vi "libera.vi"() -> ()   [LabVIEW 2014]
uses:
  chaos-common-crest/LabVIEW/LV14/chaosui-crest/VIs/ChaosDevState.ctl
  <vilib>/Utility/file.llb/Write To Spreadsheet File (I64).vi
  chaos-common-crest/LabVIEW/LV14/chaosui-crest/chaosui-crest.lvlib
panel:
  in  "DataFile":path
  out "libera_error":i32
  out "STATUS":string
  out "SA_OUT":T1(array[cluster])
  out "ADC_CW":T2(array[cluster])
  out "AVG_OUT":cluster{"AVG":i32}[](array[cluster])
  out "ADC_SP":T3(array[cluster])
  in  "AVG":bool=TRUE
  in  "STATE":bool=TRUE
  in  "stop":bool
  in  "loops":i32=10
  in  "DECIMATED":bool
  out "DD_OUT":T4(array[cluster])
  in  "refresh (ms)":u32=200
  out "samples":i32
  out "mode":i32
  out "Device State":T5
  out "nok":i32
  out "dev_error":bool
  out "acquisitions":u64
  out "timestamp":u64
  in  "Samples":u32=10
  in  "TRIGGERED":bool
  in  "ADC CW":bool
  in  "ADC SP":bool
  in  "SA":bool
  in  "DD":bool
  in  "!CHAOS URL":string="chaost-webui1.chaos.lnf.infn.it:8081"
  in  "LiberaID":string="LIBERA02/LIBERA_ACQUIRE0"
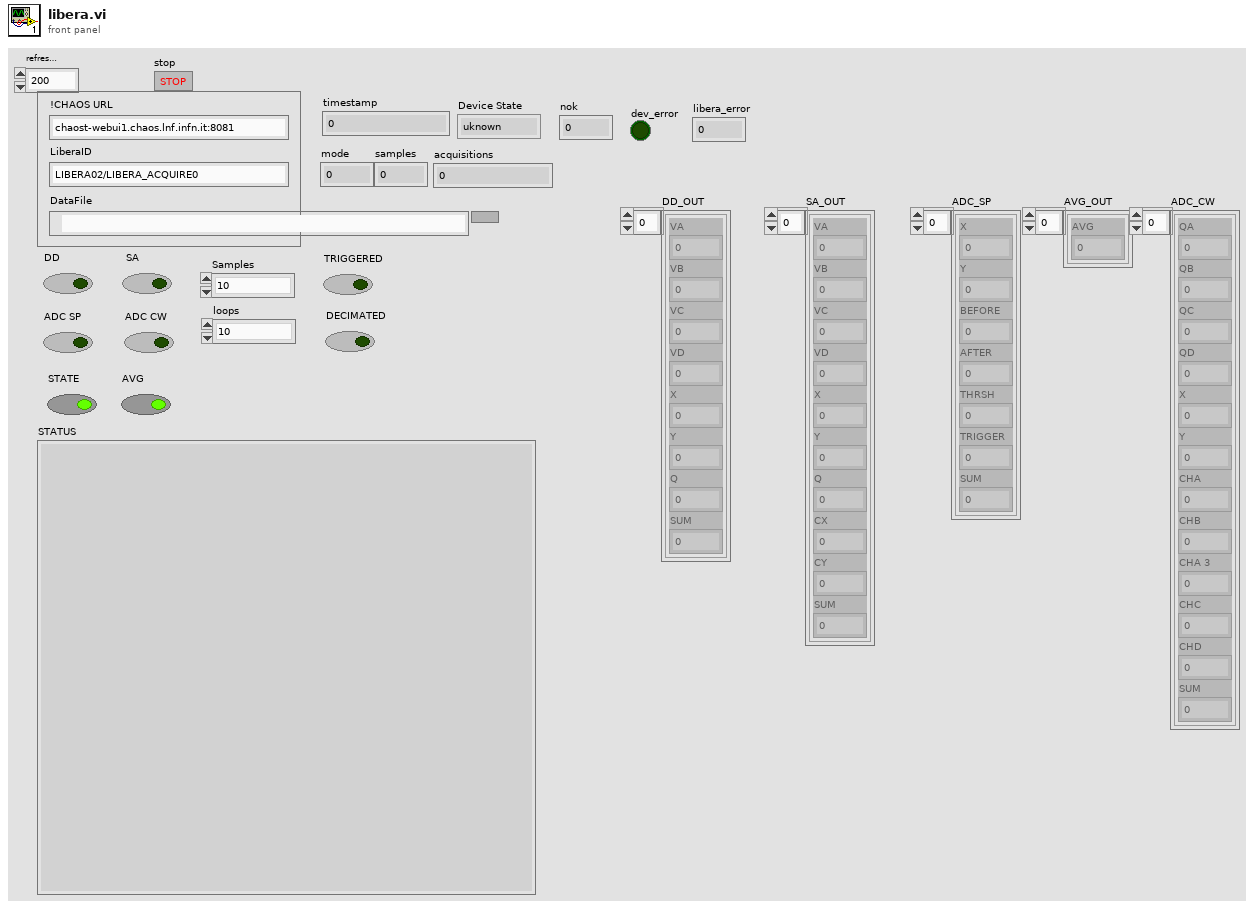
[diagram p1: front panel]
types:
  T1 = cluster{"VA":i32, "VB":i32, "VC":i32, "VD":i32, "X":i32, "Y ":i32, "Q":i32, "CX":i32, "CY":i32, "SUM":i32}[]
  T2 = cluster{"QA":i32, "QB":i32, "QC":i32, "QD":i32, "X":i32, "Y":i32, "CHA":i32, "CHB":i32, "CHA 3":i32, "CHC":i32, "CHD":i32, "SUM":i32}[]
  T3 = cluster{"X":i32, "Y":i32, "BEFORE":i32, "AFTER":i32, "THRSH":i32, "TRIGGER":i32, "SUM":i32}[]
  T4 = cluster{"VA":i32, "VB":i32, "VC":i32, "VD":i32, "X":i32, "Y ":i32, "Q":i32, "SUM":i32}[]
  T5 = typedef "ChaosDevState.ctl" = enum16{"uknown", "stop", "init", "deinit", "start"}
  T6 = typedef "LabVIEWHTTPClient.lvlib/ClientHandle.ctl" = refnum<k1>
  T7 = cluster{"client handle out":T6, "chaoswanurl":string}
  T8 = enum16{"stopAcquire", "setTime", "acquireAVG", "acquireADCSP", "acquireADCCW", "acquireStream", "acquireDD"}
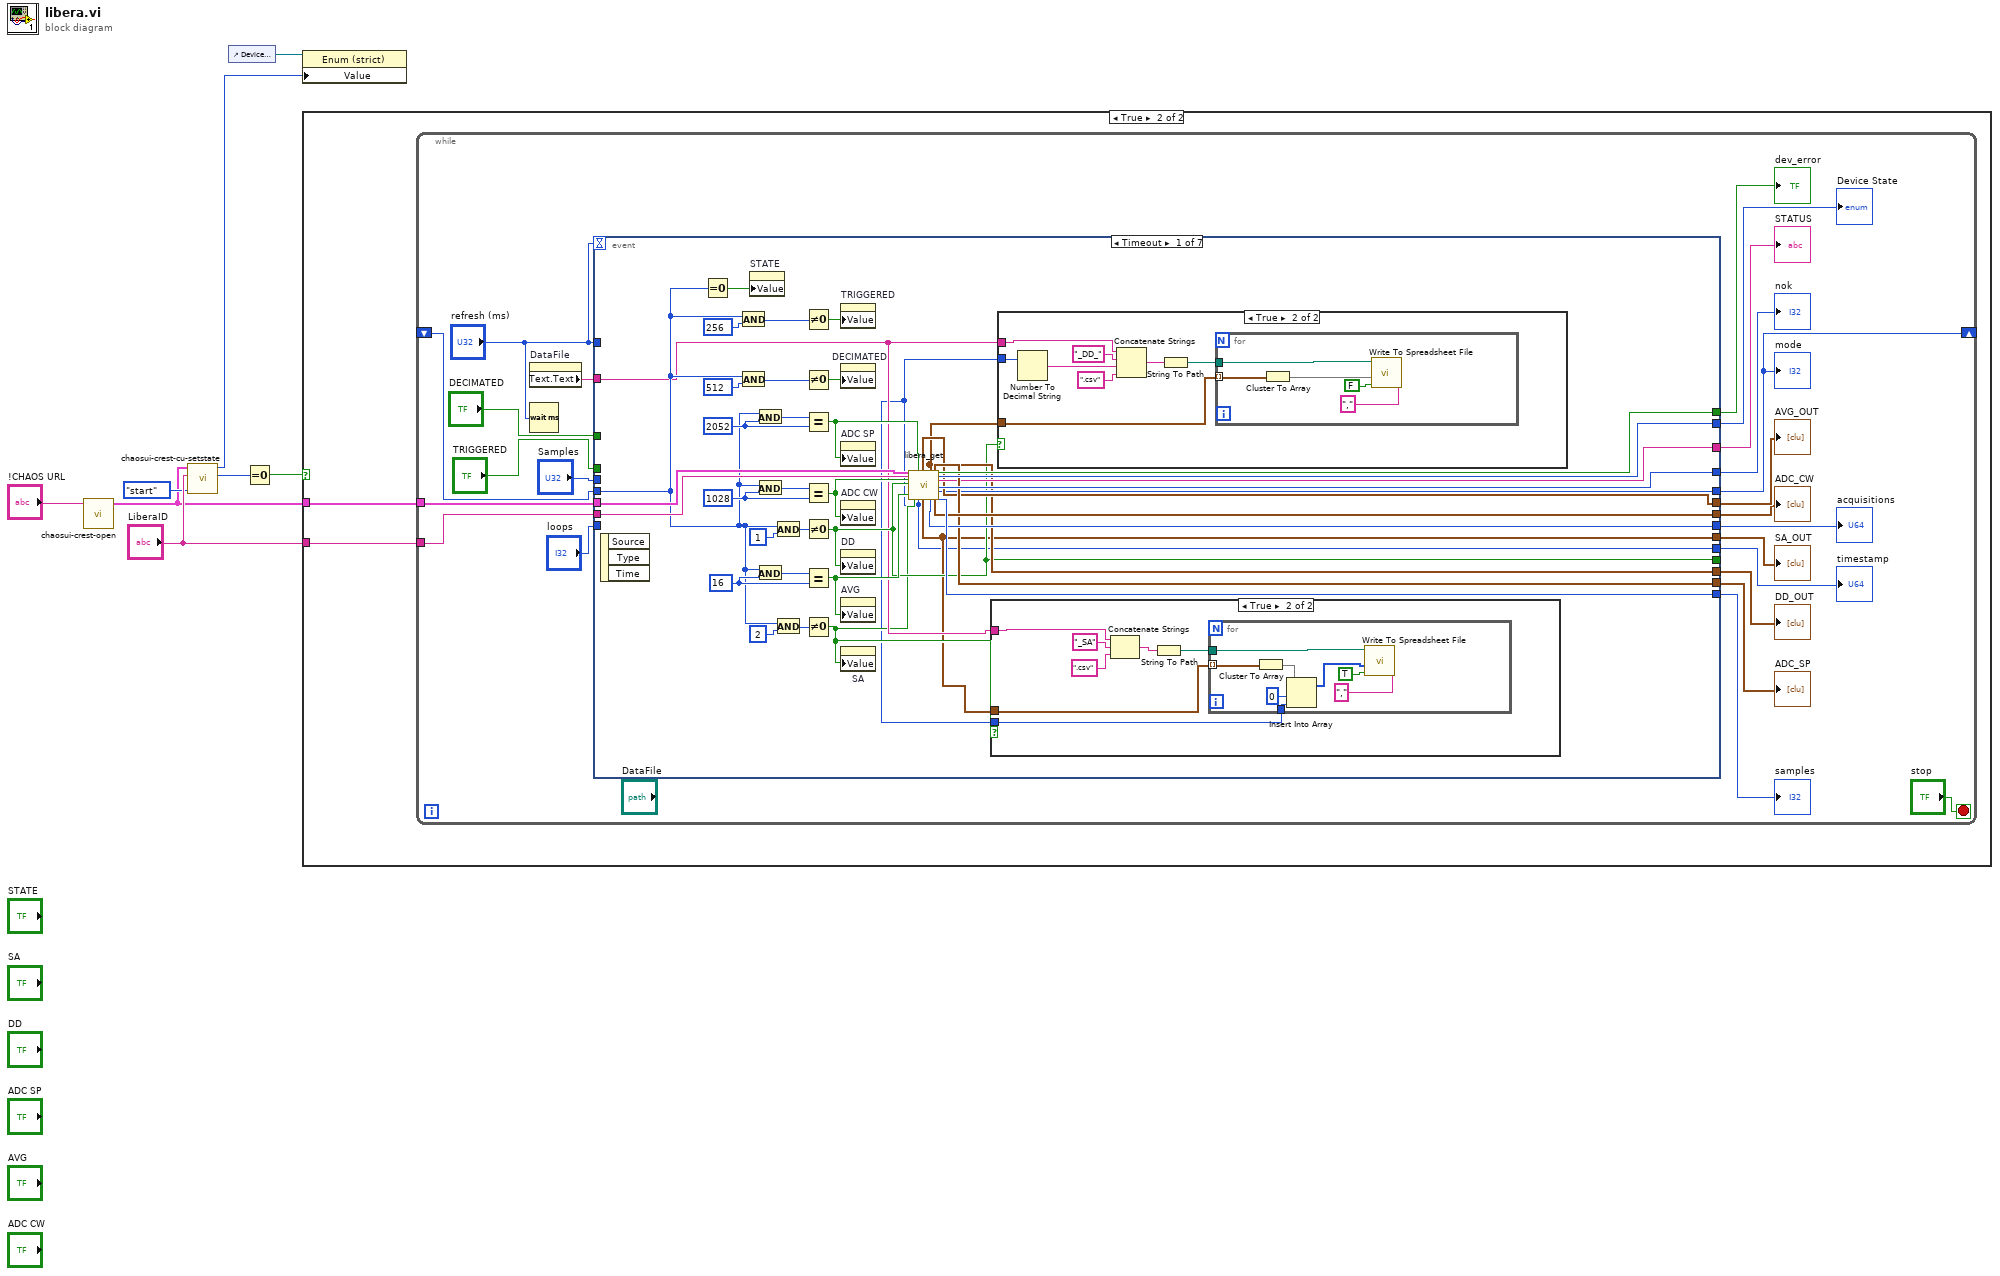
[diagram p0: block diagram]
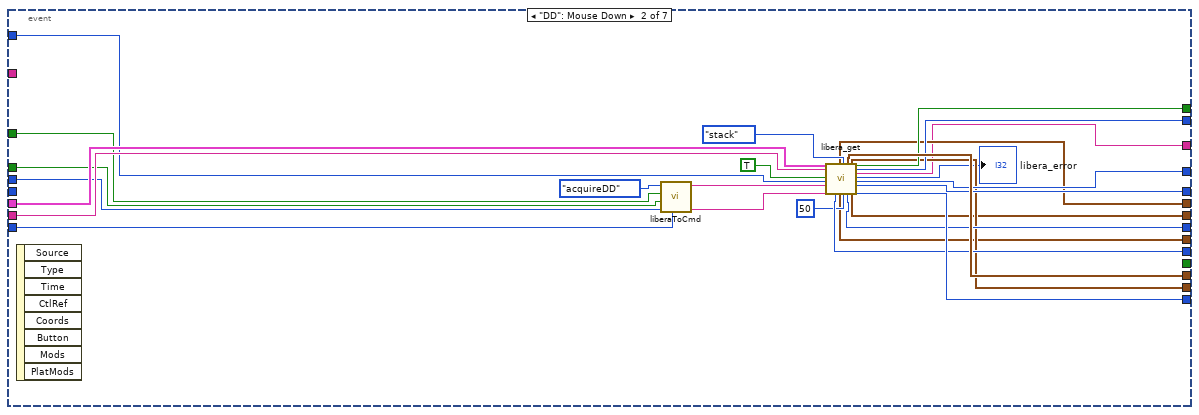
[diagram p5: hidden frame]
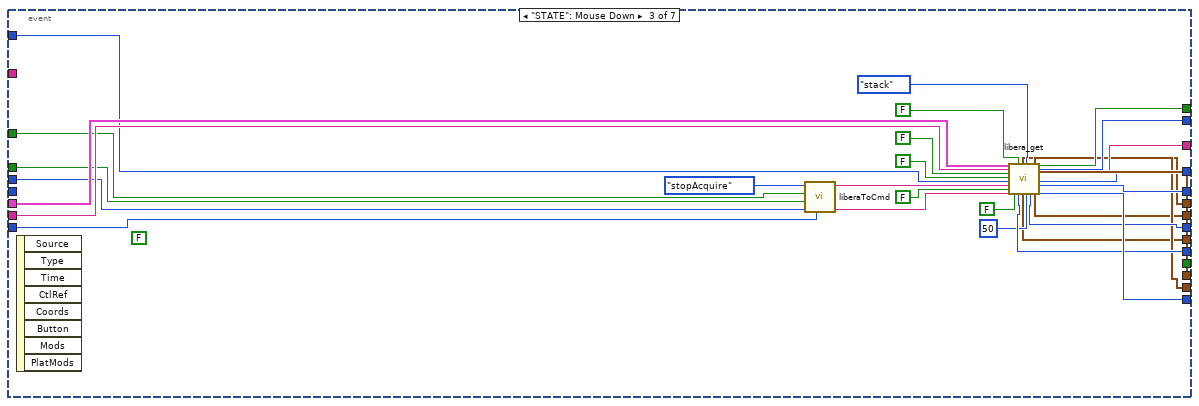
[diagram p6: hidden frame]
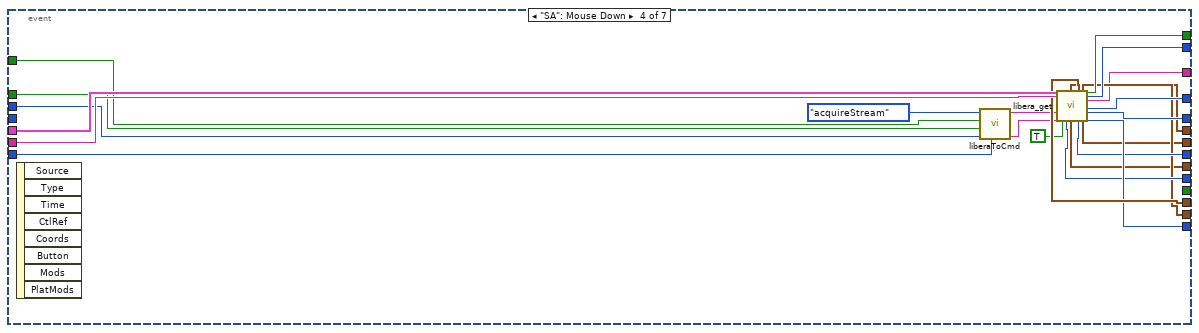
[diagram p7: hidden frame]
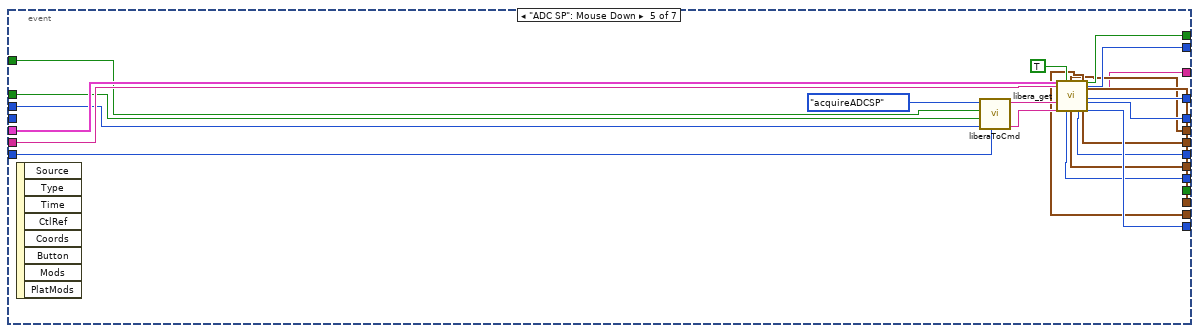
[diagram p8: hidden frame]
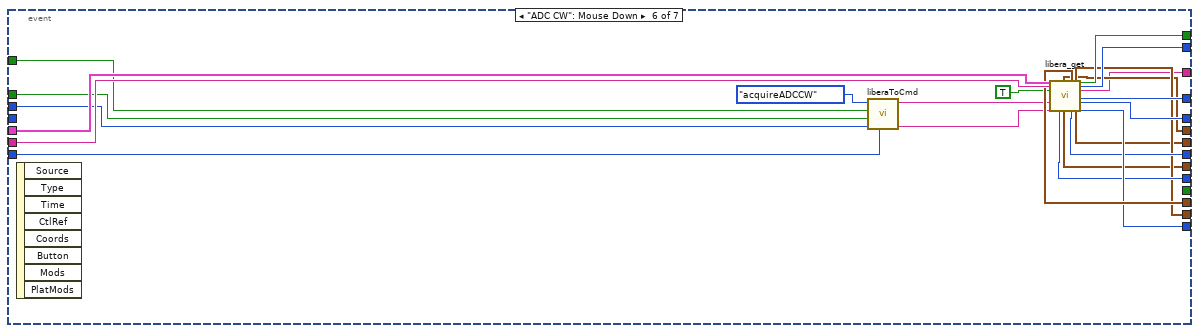
[diagram p9: hidden frame]
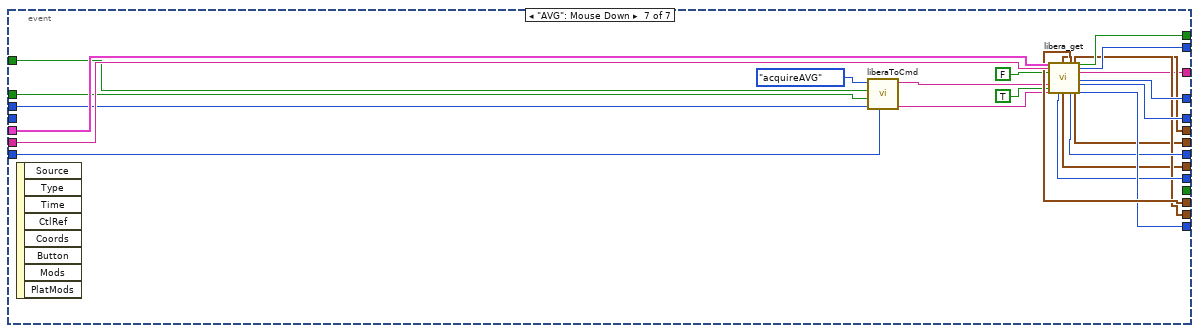
[diagram p10: hidden frame]
diagram:
  n1 = call "chaosui-crest-open.vi"("chaoswanurl"="!CHAOS URL") -> ("handle"=w1:T7)  [unwired: 10 in]
  n2 = call "chaosui-crest-cu-setstate.vi"("dev_state"=ChaosDevState."start", "cuname"="LiberaID", "handleConnection"=w1) -> ("nok"=w3:i32, "dev_state_out"=w4:T5)  [unwired: 1 in, 3 out]
  n3 = control-ref of="Device State"() -> (w5:refnum<vi>)
  n4 = Equal To 0?(x=w3) -> (x = 0?=w7:bool)
  n5 = property class="Enum (strict)"(reference=w5, "Value"=w4) -> ()  [unwired: 1 in, 2 out]
  n6 = case shown="True" w7 {
    tunnel: w1 -> [_ w10]
    tunnel: "LiberaID" -> [_ w9]
    frame False {
    }
    frame True {
      n7 = while {
        tunnel: w10 -> [w22]
        tunnel: w9 -> [w21]
        shift-right: [w20] -> _
        shift-left: _ -> [w19]
        stop <- "stop" stop-if-true
        n8 = property on="DataFile" class="Path"() -> ("Text.Text"=w11:string)  [unwired: 2 in, 2 out]
        n9 = Wait (ms)(milliseconds to wait="refresh (ms)") -> ()  [unwired: 1 out]
        n10 = event shown="[0] Timeout" {
          selector: _ -> [_ _ _ _ _ _ _]
          dyn-events: _ -> [_ _ _ _ _ _ _]
          timeout: "refresh (ms)" -> [_ _ _ _ _ _ _]
          tunnel: w22 -> [w72 w127 w157 w180 w203 w226 w250]
          tunnel: w21 -> [w71 w126 w156 w179 w202 w225 w249]
          tunnel: [w70 w124 w154 w177 w200 w223 w247] -> w33
          tunnel: [w69 w123 w153 w176 w199 w222 w246] -> w32
          tunnel: [w68 w122 w152 w175 w198 w221 w245] -> w31
          tunnel: [w40 w121 w151 w174 w197 w220 w244] -> w20
          tunnel: [w67 w120 w150 w173 w196 w219 w243] -> w30
          tunnel: [w66 w119 w149 w172 w195 w218 w242] -> w29
          tunnel: [w34 w118 w148 w171 w194 w217 w241] -> w12
          tunnel: [w39 w125 w155 w178 w201 w224 w248] -> w13
          tunnel: "Samples" -> [_ w117 w147 w170 w193 w216 w240]
          tunnel: "TRIGGERED" -> [_ w116 w146 w169 w192 w215 w239]
          tunnel: "DECIMATED" -> [_ w115 w145 w168 w191 w214 w238]
          tunnel: "loops" -> [_ w112 w142 w164 w187 w210 w234]
          tunnel: "refresh (ms)" -> [_ w110 w140 _ _ _ _]
          tunnel: w19 -> [w46 _ _ _ _ _ _]
          tunnel: [w43 w106 w131 w162 w185 w208 w231] -> w18
          tunnel: [w41 w105 w130 w161 w184 w207 w230] -> w17
          tunnel: [w44 w103 w129 w158 w182 w205 w229] -> w16
          tunnel: [w35 w102 w128 w159 w181 w204 w228] -> w15
          tunnel: [w42 w104 w132 w160 w183 w206 w227] -> w14
          tunnel: [w38 _ _ _ _ _ _] -> _
          tunnel: w11 -> [w37 _ _ _ _ _ _]
          event Timeout {
            w53 = u32 16 ("y")
            w57 = u32 1028 ("y")
            w59 = u32 2052 ("y")
            n11 = event-data() -> ()  [unwired: 1 in, 3 out]
            n12 = Equal To 0?(x=w46) -> (x = 0?=w63:bool)
            n13 = And(x=w46, y=u32 256) -> (x .and. y?=w51:u32)
            n14 = And(x=w46, y=u32 512) -> (x .and. y?=w47:u32)
            n15 = property on="STATE" class="Bool (strict)"("Value"=w63) -> ()  [unwired: 2 in, 2 out]
            n16 = And(x=w46, y=w59) -> (x .and. y?=w60:u32)
            n17 = And(x=w46, y=w57) -> (x .and. y?=w56:u32)
            n18 = And(x=w46, y=w53) -> (x .and. y?=w54:u32)
            n19 = And(x=w46, y=u32 1) -> (x .and. y?=w64:u32)
            n20 = And(x=w46, y=u32 2) -> (x .and. y?=w61:u32)
            n21 = Not Equal To 0?(x=w51) -> (x != 0?=w49:bool)
            n22 = Not Equal To 0?(x=w47) -> (x != 0?=w45:bool)
            n23 = Equal?(x=w60, y=w59) -> (x = y?=w58:bool)
            n24 = Equal?(x=w56, y=w57) -> (x = y?=w55:bool)
            n25 = Not Equal To 0?(x=w64) -> (x != 0?=w38:bool)
            n26 = Equal?(x=w54, y=w53) -> (x = y?=w52:bool)
            n27 = Not Equal To 0?(x=w61) -> (x != 0?=w36:bool)
            n28 = property on="TRIGGERED" class="Bool (strict)"("Value"=w49) -> ()  [unwired: 2 in, 2 out]
            n29 = property on="DECIMATED" class="Bool (strict)"("Value"=w45) -> ()  [unwired: 2 in, 2 out]
            n30 = property on="ADC SP" class="Bool (strict)"("Value"=w58) -> ()  [unwired: 2 in, 2 out]
            n31 = property on="ADC CW" class="Bool (strict)"("Value"=w55) -> ()  [unwired: 2 in, 2 out]
            n32 = property on="DD" class="Bool (strict)"("Value"=w38) -> ()  [unwired: 2 in, 2 out]
            n33 = property on="AVG" class="Bool (strict)"("Value"=w52) -> ()  [unwired: 2 in, 2 out]
            n34 = property on="SA" class="Bool (strict)"("Value"=w36) -> ()  [unwired: 2 in, 2 out]
            n35 = call "libera_get.vi"("handleConnection"=w72, "cuname"=w71, "Enable ADC CW"=w55, "Enable DD"=w38, "Enable AVG"=w52, "Enable SA"=w36, "Enable ADC SP"=w58) -> ("timestamp"=w34:u64, "AVG"=w41:cluster{"AVG":i32}[], "SA"=w35:T1, "DD"=w39:T4, "acquisitions"=w66:u64, "ADC_SP"=w43:T3, "ADC_CW"=w44:T2, "dev_error"=w70:bool, "dev_state"=w69:T5, "STATUS"=w42:string, "nok"=w68:i32, "mode"=w40:i32, "samples"=w67:i32)  [unwired: 7 in, 1 out]
            n36 = case shown="True" w36 {
              tunnel: w35 -> [_ w77]
              tunnel: w37 -> [_ w76]
              tunnel: w34 -> [_ w73]
              frame False {
              }
              frame True {
                n37 = Concatenate Strings(w76, "_SA" ("string"), ".csv" ("name or relative path")) -> (w75:string)
                n38 = String To Path(string=w75) -> (path=w74:path)
                n39 = for {
                  tunnel: w74 -> [w87]
                  tunnel: w77 -> [w86] mode=indexing
                  tunnel: w73 -> [w81]
                  n40 = Cluster To Array(cluster=w86) -> (array=w83:i32[])
                  n41 = Insert Into Array(array=w83, index=0, new element=w81) -> (w80:i32[])
                  n42 = call-poly <vilib>:"Write To Spreadsheet File.vi"("delimiter (\\t)"="," ("delimiter (\\t)"), "append to file? (new file:F)"=TRUE, "1D data"=w80, "file path (dialog if empty)"=w87) -> ()  [unwired: 4 in, 1 out]
                }
              }
            }
            n43 = case shown="True" w38 {
              tunnel: w34 -> [_ w95]
              tunnel: w39 -> [_ w91]
              tunnel: w37 -> [_ w90]
              frame False {
              }
              frame True {
                n44 = Number To Decimal String(number=w95) -> (decimal integer string=w94:string)  [unwired: 1 in]
                n45 = Concatenate Strings(w90, "_DD_" ("string"), w94, ".csv" ("name or relative path")) -> (w89:string)
                n46 = String To Path(string=w89) -> (path=w88:path)
                n47 = for {
                  tunnel: w88 -> [w100]
                  tunnel: w91 -> [w99] mode=indexing
                  n48 = Cluster To Array(cluster=w99) -> (array=w98:i32[])
                  n49 = call-poly <vilib>:"Write To Spreadsheet File.vi"("delimiter (\\t)"="," ("delimiter (\\t)"), "append to file? (new file:F)"=FALSE, "1D data"=w98, "file path (dialog if empty)"=w100) -> ()  [unwired: 4 in, 1 out]
                }
              }
            }
          }
          event "DD": Mouse Down {
            n50 = event-data() -> ()  [unwired: 1 in, 8 out]
            n51 = call "liberaToCmd.vi"("loops"=w112, "samples"=w117, "triggered"=w116, "decimated"=w115, "cmd"=T8."acquireDD") -> ("jsonargs"=w113:string, "cmd"=w114:string)  [unwired: 5 in]
            n52 = call "libera_get.vi"("handleConnection"=w127, "cuname"=w126, "Enable DD"=TRUE, "sched (ms)"=w110, "cmd"=w114, "args"=w113, "cmd submission mode"=enum16{"stack", "kill previous"}."stack", "prio"=50) -> ("timestamp"=w118:u64, "AVG"=w105:cluster{"AVG":i32}[], "SA"=w102:T1, "DD"=w125:T4, "acquisitions"=w119:u64, "ADC_SP"=w106:T3, "ADC_CW"=w103:T2, "dev_error"=w124:bool, "dev_state"=w123:T5, "STATUS"=w104:string, "libera_error"=→"libera_error":i32, "nok"=w122:i32, "mode"=w121:i32, "samples"=w120:i32)  [unwired: 6 in]
          }
          event "STATE": Mouse Down {
            (unwired) FALSE ("Enable SA")
            n53 = event-data() -> ()  [unwired: 1 in, 8 out]
            n54 = call "liberaToCmd.vi"("loops"=w142, "samples"=w147, "triggered"=w146, "decimated"=w145, "cmd"=T8."stopAcquire") -> ("jsonargs"=w143:string, "cmd"=w144:string)  [unwired: 5 in]
            n55 = call "libera_get.vi"("handleConnection"=w157, "cuname"=w156, "Enable ADC CW"=FALSE, "Enable DD"=FALSE, "sched (ms)"=w140, "cmd"=w144, "Enable AVG"=FALSE, "args"=w143, "Enable SA"=FALSE, "Enable ADC SP"=FALSE, "cmd submission mode"=enum16{"stack", "kill previous"}."stack", "prio"=50) -> ("timestamp"=w148:u64, "AVG"=w130:cluster{"AVG":i32}[], "SA"=w128:T1, "DD"=w155:T4, "acquisitions"=w149:u64, "ADC_SP"=w131:T3, "ADC_CW"=w129:T2, "dev_error"=w154:bool, "dev_state"=w153:T5, "STATUS"=w132:string, "nok"=w152:i32, "mode"=w151:i32, "samples"=w150:i32)  [unwired: 2 in, 1 out]
          }
          event "SA": Mouse Down {
            n56 = event-data() -> ()  [unwired: 1 in, 8 out]
            n57 = call "liberaToCmd.vi"("loops"=w164, "samples"=w170, "triggered"=w169, "decimated"=w168, "cmd"=T8."acquireStream") -> ("jsonargs"=w165:string, "cmd"=w166:string)  [unwired: 5 in]
            n58 = call "libera_get.vi"("handleConnection"=w180, "cuname"=w179, "cmd"=w166, "args"=w165, "Enable SA"=TRUE) -> ("timestamp"=w171:u64, "AVG"=w161:cluster{"AVG":i32}[], "SA"=w159:T1, "DD"=w178:T4, "acquisitions"=w172:u64, "ADC_SP"=w162:T3, "ADC_CW"=w158:T2, "dev_error"=w177:bool, "dev_state"=w176:T5, "STATUS"=w160:string, "nok"=w175:i32, "mode"=w174:i32, "samples"=w173:i32)  [unwired: 9 in, 1 out]
          }
          event "ADC SP": Mouse Down {
            n59 = event-data() -> ()  [unwired: 1 in, 8 out]
            n60 = call "liberaToCmd.vi"("loops"=w187, "samples"=w193, "triggered"=w192, "decimated"=w191, "cmd"=T8."acquireADCSP") -> ("jsonargs"=w188:string, "cmd"=w189:string)  [unwired: 5 in]
            n61 = call "libera_get.vi"("handleConnection"=w203, "cuname"=w202, "cmd"=w189, "args"=w188, "Enable ADC SP"=TRUE) -> ("timestamp"=w194:u64, "AVG"=w184:cluster{"AVG":i32}[], "SA"=w181:T1, "DD"=w201:T4, "acquisitions"=w195:u64, "ADC_SP"=w185:T3, "ADC_CW"=w182:T2, "dev_error"=w200:bool, "dev_state"=w199:T5, "STATUS"=w183:string, "nok"=w198:i32, "mode"=w197:i32, "samples"=w196:i32)  [unwired: 9 in, 1 out]
          }
          event "ADC CW": Mouse Down {
            n62 = event-data() -> ()  [unwired: 1 in, 8 out]
            n63 = call "liberaToCmd.vi"("loops"=w210, "samples"=w216, "triggered"=w215, "decimated"=w214, "cmd"=T8."acquireADCCW") -> ("jsonargs"=w211:string, "cmd"=w212:string)  [unwired: 5 in]
            n64 = call "libera_get.vi"("handleConnection"=w226, "cuname"=w225, "Enable ADC CW"=TRUE, "cmd"=w212, "args"=w211) -> ("timestamp"=w217:u64, "AVG"=w207:cluster{"AVG":i32}[], "SA"=w204:T1, "DD"=w224:T4, "acquisitions"=w218:u64, "ADC_SP"=w208:T3, "ADC_CW"=w205:T2, "dev_error"=w223:bool, "dev_state"=w222:T5, "STATUS"=w206:string, "nok"=w221:i32, "mode"=w220:i32, "samples"=w219:i32)  [unwired: 9 in, 1 out]
          }
          event "AVG": Mouse Down {
            n65 = event-data() -> ()  [unwired: 1 in, 8 out]
            n66 = call "liberaToCmd.vi"("loops"=w234, "samples"=w240, "triggered"=w239, "decimated"=w238, "cmd"=T8."acquireAVG") -> ("jsonargs"=w235:string, "cmd"=w236:string)  [unwired: 5 in]
            n67 = call "libera_get.vi"("handleConnection"=w250, "cuname"=w249, "Enable ADC CW"=FALSE, "cmd"=w236, "Enable AVG"=TRUE, "args"=w235) -> ("timestamp"=w241:u64, "AVG"=w230:cluster{"AVG":i32}[], "SA"=w228:T1, "DD"=w248:T4, "acquisitions"=w242:u64, "ADC_SP"=w231:T3, "ADC_CW"=w229:T2, "dev_error"=w247:bool, "dev_state"=w246:T5, "STATUS"=w227:string, "nok"=w245:i32, "mode"=w244:i32, "samples"=w243:i32)  [unwired: 8 in, 1 out]
          }
        }
        "timestamp" <- w12
        "acquisitions" <- w29
        "dev_error" <- w33
        "nok" <- w31
        "Device State" <- w32
        "mode" <- w20
        "samples" <- w30
        "DD_OUT" <- w13
        "ADC_SP" <- w18
        "AVG_OUT" <- w17
        "ADC_CW" <- w16
        "SA_OUT" <- w15
        "STATUS" <- w14
      }
    }
  }
